vi "ResonanceAnalyzer.vi"() -> ()   [LabVIEW 2015]
uses:
  <vilib>/imath/engines/lvmath2/RunTimeEngine/Managers/WorkSpace/UID Generator.vi
  <vilib>/imath/engines/lvmath2/RunTimeEngine/RangeToken/NIMS_Range.vi
  <instcachedir>/0/NIMS_Range_D919CC09935940E88F755EC1C6F49AC1.lvgen/NIMS_Range_D919CC09935940E88F755EC1C6F49AC1_000.vi
  <vilib>/imath/engines/lvmath2/RunTimeEngine/RunTimeType/NIMS_RunTimeType_From StrictType (excl LVString).vi
  <instcachedir>/0/NIMS_RunTimeType_From StrictType (excl LVString)_EB1C38A9BC5048DA9ABDA8F781E54D21.lvgen/NIMS_RunTimeType_From StrictType (excl LVString)_EB1C38A9BC5048DA9ABDA8F781E54D21_000.vi
  <vilib>/imathl/engines/lvmath/Functions/Error Handling/Create Error.vi
  <vilib>/imath/engines/lvmath2/RunTimeEngine/LocalVariableDefStatement/MC_LocalVariableDefStatement_Display.vi
  <vilib>/imath/engines/lvmath2/RunTimeEngine/Managers/SymbolTable/Clear UID.vi
  <vilib>/imath/engines/lvmath2/RunTimeEngine/NodeEndStatement/NIMS_NodeEndStatement_Output.vi
  <instcachedir>/0/NIMS_NodeEndStatement_Output_53EC0D466D134D7ABD903AC30B43404B.lvgen/NIMS_NodeEndStatement_Output_53EC0D466D134D7ABD903AC30B43404B_005.vi
  <vilib>/imath/engines/lvmath2/RunTimeEngine/ErrorHandling/NIMS_Finalize Error.vi
  <vilib>/Utility/file.llb/Read Delimited Spreadsheet (DBL).vi
  <vilib>/imath/engines/lvmath2/RunTimeEngine/Managers/SymbolTable/NIMS_WorkSpace.lvlib
panel:
  out "XY Graph":cluster{"all rows":dbl[], "all rows":dbl[]}(graph)
  in  "Tab Control":enum32{" Simulation", "Experiment"}(tab)
  in  "Cluster":T1
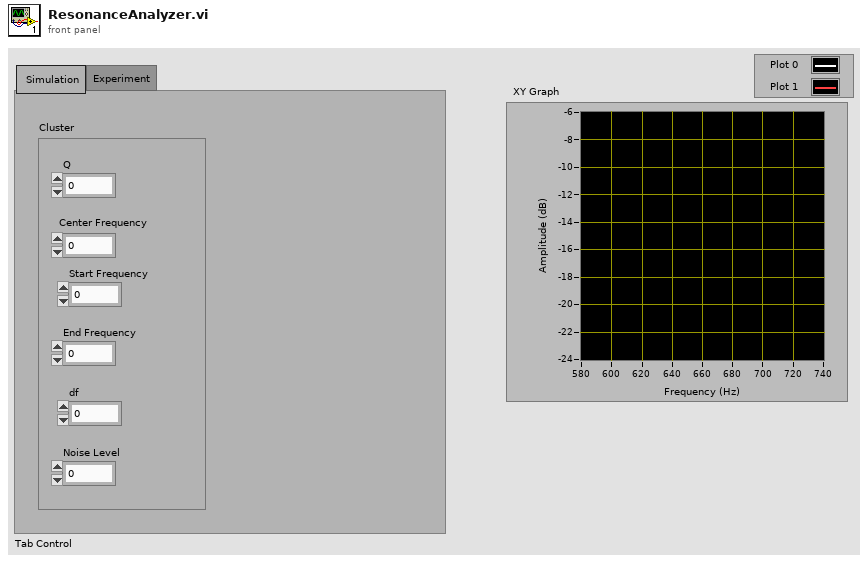
[diagram p1: front panel]
types:
  T1 = cluster{"Q":dbl, "Center Frequency":dbl, "Start Frequency":dbl, "End Frequency":dbl, "df ":dbl, "Noise Level":dbl}
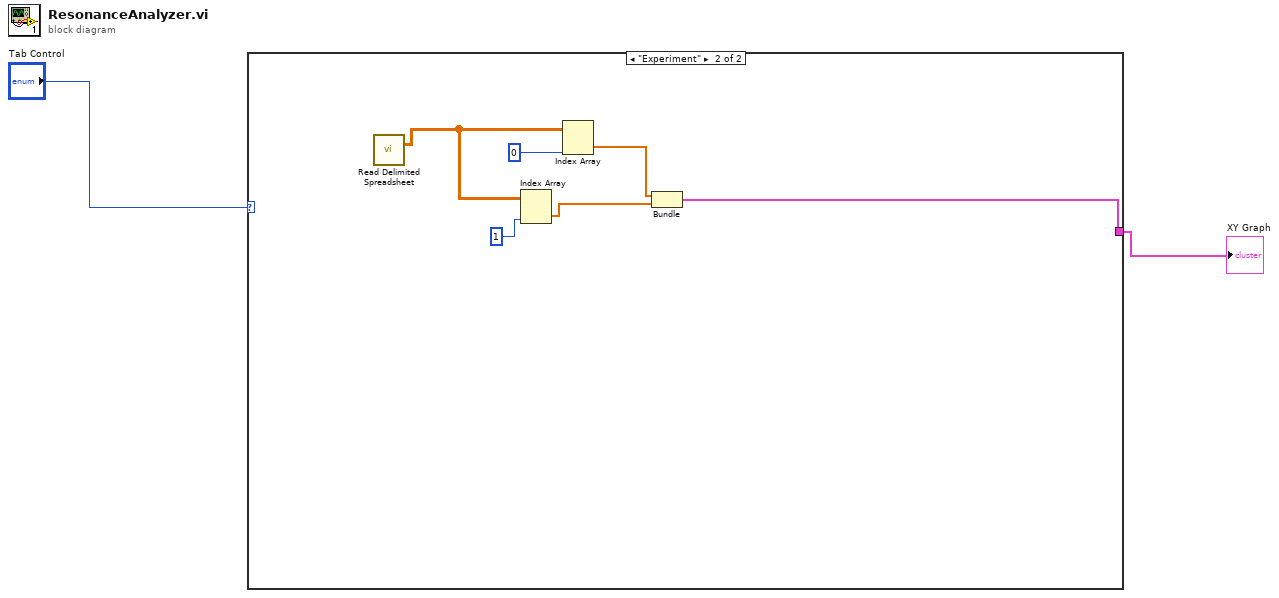
[diagram p0: block diagram]
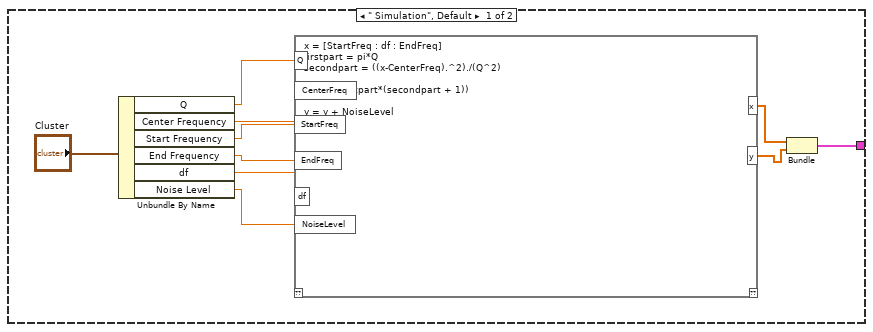
[diagram p2: hidden frame]
diagram:
  n1 = case shown="\"Experiment\"" "Tab Control" {
    tunnel: [w3 w139] -> w1
    frame " Simulation", Default {
      n2 = Unbundle By Name("Cluster") -> ("Q"=w11:dbl, "Center Frequency"=w10:dbl, "Start Frequency"=w9:dbl, "End Frequency"=w8:dbl, "df"=w7:dbl, "Noise Level"=w6:dbl)
      n3 = mathscript code="x = [StartFreq : df : EndFreq]\nfirstpart = pi*Q\nsecondpart = ((x-CenterFreq).^2)./(Q^2)\n\ny = 1./(firstpart*(secondpart + 1))\n\ny = y + NoiseLevel"("Q"=w11, "CenterFreq"=w10, "StartFreq"=w9, "EndFreq"=w8, "df"=w7, "NoiseLevel"=w6) -> ("y"=w4:dbl[], "x"=w5:dbl[])  [unwired: 1 in, 1 out]
      n4 = Bundle("x"=w5, "y"=w4) -> (w3:cluster{"x":dbl[], "y":dbl[]})  [unwired: 1 in]
    }
    frame "Experiment" {
      n5 = call-poly <vilib>:"Read Delimited Spreadsheet.vi"() -> ("all rows"=w142:dbl[][])  [unwired: 10 in, 5 out]
      n6 = Index Array(array=w142, index (col)=1) -> (element=w140:dbl[])  [unwired: 1 in]
      n7 = Index Array(array=w142, index (col)=0) -> (element=w141:dbl[])  [unwired: 1 in]
      n8 = Bundle("all rows"=w141, "all rows"=w140) -> (w139:cluster{"all rows":dbl[], "all rows":dbl[]})  [unwired: 1 in]
    }
  }
  "XY Graph" <- w1
